vi "Get Image Size (Pixels).vi"(8 "Error In":errorcluster) -> (0 "Error Out":errorcluster, 2 "Columns (Pixels)":i32, 3 "Rows (Pixels)":i32)   [LabVIEW 2018, in "Image Management.lvlib"]
uses:
  Image Management.lvlib
  Action.ctl
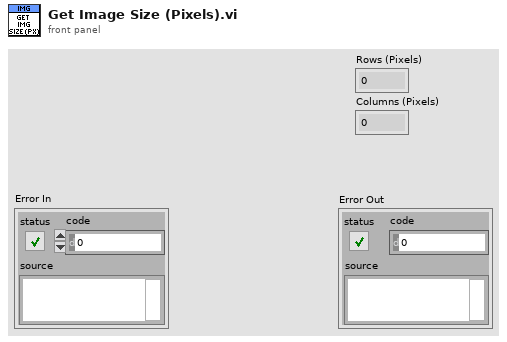
[diagram p1: front panel]
types:
  T1 = typedef "Image Management.lvlib/Action.ctl" = enum16{"Init", "Open Image in Default Program", "Find Linespaces", "Get Image Size (pixels)", "Close"}
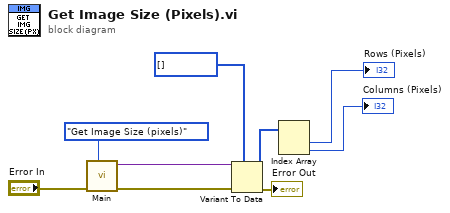
[diagram p0: block diagram]
diagram:
  n1 = call "Main.vi"("Action"=Action."Get Image Size (pixels)", "Error In"="Error In") -> ("Error Out"=w7:errorcluster, "Output"=w8:variant)  [unwired: 8 in]
  n2 = Variant To Data(error in=w7, type=i32[] [] ("appended array"), Variant=w8) -> (data=w6:i32[], error out=→"Error Out":errorcluster)
  n3 = Index Array(array=w6) -> (element #1=→"Rows (Pixels)":i32, element #2=→"Columns (Pixels)":i32)  [unwired: 2 in]
